vi "CheckforLiveConnections.vi"(2 "Node URI":string, 3 "topic":string, 4 "Connections":T1(array[cluster])) -> (0 "Connection":T2, 1 "new?":bool)   [LabVIEW 2016]
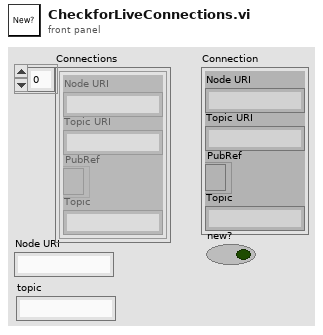
[diagram p1: front panel]
types:
  T1 = cluster{"Node URI":string, "Topic URI":string, "PubRef":refnum<k5>, "Topic":string}[]
  T2 = cluster{"Node URI":string, "Topic URI":string, "PubRef":refnum<k5>, "Topic":string}
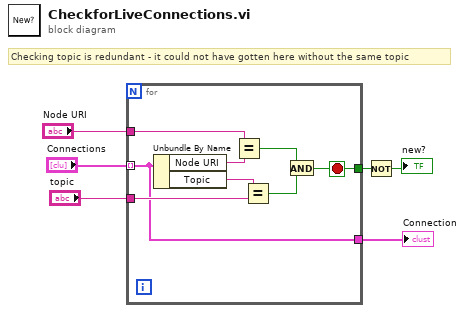
[diagram p0: block diagram]
diagram:
  # "Checking topic is redundant - it could not have gotten here without the same topic"
  n1 = for {
    tunnel: "Connections" -> [w7] mode=indexing
    tunnel: "Node URI" -> [w13]
    tunnel: "topic" -> [w11]
    tunnel: [w8] -> w3
    tunnel: [w7] -> w2
    stop <- w8 stop-if-true
    n2 = Unbundle By Name(w7) -> ("Node URI"=w14:string, "Topic"=w12:string)
    n3 = Equal?(x=w13, y=w14) -> (x = y?=w10:bool)
    n4 = Equal?(x=w12, y=w11) -> (x = y?=w9:bool)
    n5 = And(x=w10, y=w9) -> (x .and. y?=w8:bool)
  }
  "Connection" <- w2
  n6 = Not(x=w3) -> (.not. x?=→"new?":bool)
